vi "OSICS_FBL_Example.vi"() -> ()   [LabVIEW 2014, in "OSICS_LIB.lvlib"]
doc: "This example VI controls an OSICS Full Band Laser (FBL) remotely.\nAll commands and queries are sent to the OSICS SWT-APC, operating in \"Full-Band\" mode.\nThe OSICS mainframe can be connected via RS232 or GPIB."
uses:
  OSICS_LIB.lvlib
panel:
  out "Busy/Idle Status":bool
  in  "stop":bool
  in  "Laser State":bool
  in  "Power Unit":bool
  in  "WL/F unit":bool
  in  "VISA":refnum<visa-resource-name>="GPIB0::10::INSTR"
  in  "WL/Frequency Value":dbl format="%#_8g"
  in  "Power Value":dbl
  # "OSICS SWT-APC Full-Band Laser Example 1.1"
  # "l/¦"
  # "P"
  # "OSICS SWT-APC: Full-Band"
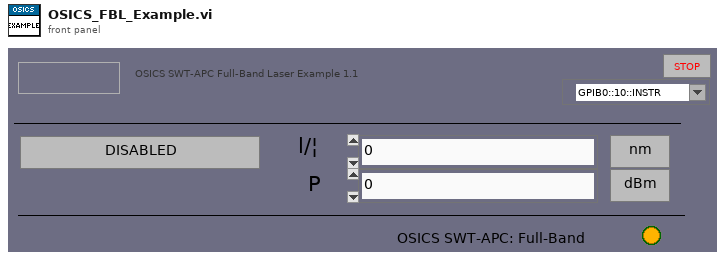
[diagram p1: front panel]
types:
  T1 = cluster{"Laser State":bool, "WL/F Value":dbl, "Power (dBm/mW)":dbl, "Power Limit":bool}
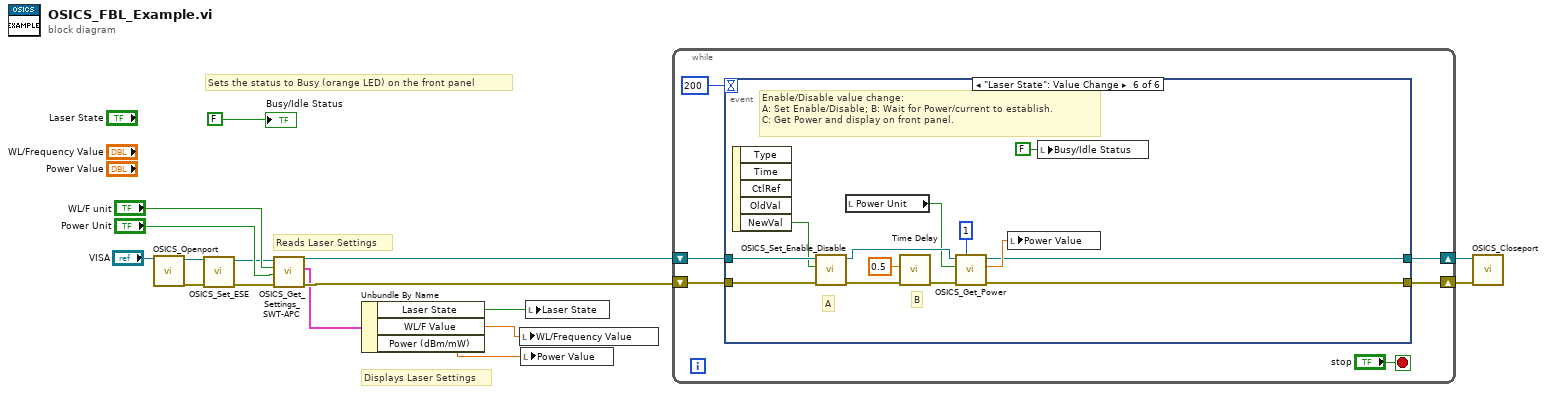
[diagram p0: block diagram]
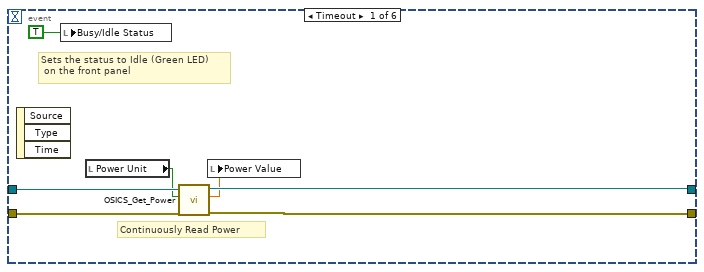
[diagram p2: hidden frame]
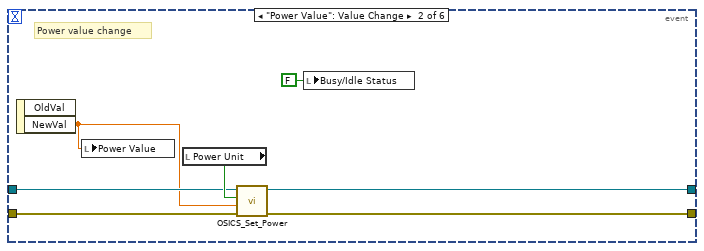
[diagram p3: hidden frame]
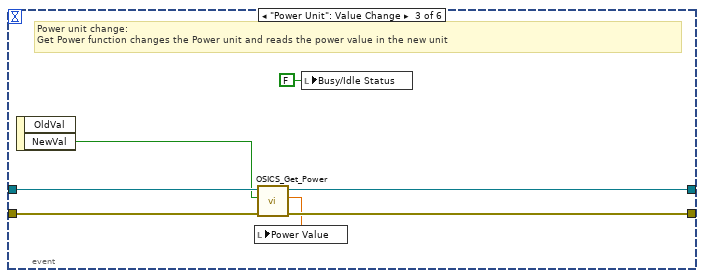
[diagram p4: hidden frame]
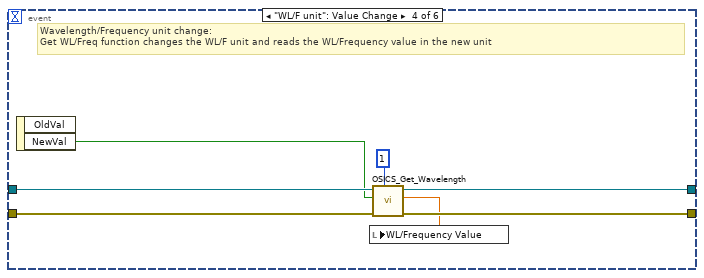
[diagram p5: hidden frame]
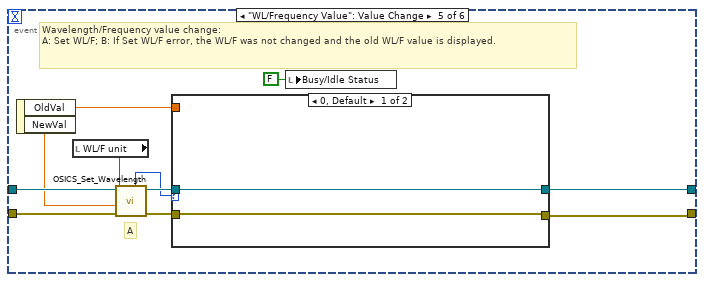
[diagram p6: hidden frame]
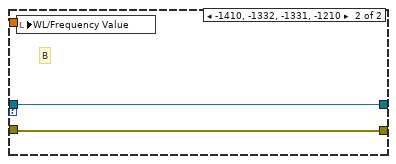
[diagram p7: hidden frame]
diagram:
  # "Sets the status to Busy (orange LED) on the front panel"
  # "Displays Laser Settings"
  # "Reads Laser Settings"
  n1 = call "OSICS_Openport.vi"("VISA IN"="VISA") -> ("error out"=w3:errorcluster, "VISA OUT"=w2:refnum<visa-resource-name>)  [unwired: 9 in]
  n2 = call "OSICS_Set_ESE.vi"("error in (no error)"=w3, "VISA resource name"=w2) -> ("error out"=w4:errorcluster, "VISA resource name out"=w1:refnum<visa-resource-name>)  [unwired: 8 in]
  n3 = call "OSICS_Get_Settings_SWT-APC.vi"("error in"=w4, "Power Unit(dBm/mW)"="Power Unit", "WL/F unit (nm/GHz)"="WL/F unit", "VISA IN"=w1) -> ("error out"=w10:errorcluster, "Laser Settings (Cluster)"=w6:T1, "VISA OUT"=w9:refnum<visa-resource-name>)  [unwired: 5 in]
  n4 = Unbundle By Name(w6) -> ("Laser State"=w11:bool, "WL/F Value"=w13:dbl, "Power (dBm/mW)"=w12:dbl)
  n5 = local write "WL/Frequency Value"(w13) -> ()
  n6 = local write "Power Value"(w12) -> ()
  n7 = local write "Laser State"(w11) -> ()
  n8 = while {
    shift-right: [w19] -> w16
    shift-left: w9 -> [w21]
    shift-right: [w18] -> w15
    shift-left: w10 -> [w20]
    stop <- "stop" stop-if-true
    n9 = event shown="[5] \"Laser State\": Value Change" {
      selector: _ -> [_ _ _ _ _ _]
      dyn-events: _ -> [_ _ _ _ _ _]
      timeout: 200 -> [_ _ _ _ _ _]
      tunnel: w21 -> [w29 w32 w43 w50 w61 w79]
      tunnel: w20 -> [w28 w33 w42 w48 w60 w78]
      tunnel: [w27 w36 w40 w46 w54 w68] -> w19
      tunnel: [w23 w34 w41 w47 w57 w70] -> w18
      event Timeout {
        # "Continuously Read Power"
        # "Sets the status to Idle (Green LED)\n on the front panel"
        n10 = event-data() -> ()  [unwired: 1 in, 3 out]
        n11 = local write "Busy/Idle Status"(TRUE ("Busy/Idle Status")) -> ()
        n12 = local read "Power Unit"() -> (w24:bool)
        n13 = call "OSICS_Get_Power.vi"("error in"=w28, "Power Unit(False: dBm)"=w24, "VISA IN"=w29) -> ("error out"=w23:errorcluster, "Power (dBm/mW)"=w25:dbl, "VISA OUT"=w27:refnum<visa-resource-name>)  [unwired: 4 in, 2 out]
        n14 = local write "Power Value"(w25) -> ()
      }
      event "Power Value": Value Change {
        # "Power value change"
        n15 = event-data() -> ("NewVal"=w30:dbl)  [unwired: 1 in, 1 out]
        n16 = local write "Power Value"(w30) -> ()
        n17 = local read "Power Unit"() -> (w35:bool)
        n18 = call "OSICS_Set_Power.vi"("error in"=w33, "P Value"=w30, "Power Unit(False:dBm)"=w35, "VISA IN"=w32) -> ("error out"=w34:errorcluster, "VISA OUT"=w36:refnum<visa-resource-name>)  [unwired: 5 in, 1 out]
        n19 = local write "Busy/Idle Status"(FALSE ("Busy/Idle Status")) -> ()
      }
      event "Power Unit": Value Change {
        # "Power unit change:\nGet Power function changes the Power unit and reads the power value in the new unit"
        n20 = event-data() -> ("NewVal"=w39:bool)  [unwired: 1 in, 1 out]
        n21 = call "OSICS_Get_Power.vi"("error in"=w42, "Power Unit(False: dBm)"=w39, "VISA IN"=w43) -> ("error out"=w41:errorcluster, "Power (dBm/mW)"=w38:dbl, "VISA OUT"=w40:refnum<visa-resource-name>)  [unwired: 4 in, 2 out]
        n22 = local write "Power Value"(w38) -> ()
        n23 = local write "Busy/Idle Status"(FALSE ("Busy/Idle Status")) -> ()
      }
      event "WL/F unit": Value Change {
        # "Wavelength/Frequency unit change:\nGet WL/Freq function changes the WL/F unit and reads the WL/Frequency value in the new unit"
        n24 = event-data() -> ("NewVal"=w49:bool)  [unwired: 1 in, 1 out]
        n25 = call "OSICS_Get_Wavelength.vi"("OSICS slot"=1, "error in"=w48, "WL/F unit (False:NM)"=w49, "VISA IN"=w50) -> ("error out"=w47:errorcluster, "WL/Frequency Value"=w45:dbl, "VISA OUT"=w46:refnum<visa-resource-name>)  [unwired: 4 in, 1 out]
        n26 = local write "WL/Frequency Value"(w45) -> ()
      }
      event "WL/Frequency Value": Value Change {
        # "A"
        # "Wavelength/Frequency value change:\nA: Set WL/F; B: If Set WL/F error, the WL/F was not changed and the old WL/F value is displayed."
        n27 = event-data() -> ("OldVal"=w58:dbl, "NewVal"=w59:dbl)  [unwired: 1 in]
        n28 = local read "WL/F unit"() -> (w53:bool)
        n29 = call "OSICS_Set_Wavelength.vi"("error in"=w60, "WL/Frequency Value"=w59, "WL/F unit (False:nm)"=w53, "VISA IN"=w61) -> ("error out"=w56:errorcluster, "VISA OUT"=w55:refnum<visa-resource-name>, "ERR"=w52:i32)  [unwired: 5 in]
        n30 = case shown="0, Default" w52 {
          tunnel: w58 -> [_ w66]
          tunnel: [w62 w65] -> w57
          tunnel: w56 -> [w62 w65]
          tunnel: w55 -> [w63 w64]
          tunnel: [w63 w64] -> w54
          frame 0, Default {
          }
          frame -1410, -1332, -1331, -1210 {
            # "B"
            n31 = local write "WL/Frequency Value"(w66) -> ()
          }
        }
        n32 = local write "Busy/Idle Status"(FALSE ("Busy/Idle Status")) -> ()
      }
      event "Laser State": Value Change {
        # "B"
        # "A"
        # "Enable/Disable value change:\nA: Set Enable/Disable; B: Wait for Power/current to establish.\nC: Get Power and display on front panel."
        n33 = event-data() -> ("NewVal"=w77:bool)  [unwired: 1 in, 4 out]
        n34 = call "OSICS_Set_Enable_Disable.vi"("error in"=w78, "Laser State (False:DISABLED)"=w77, "VISA IN"=w79) -> ("error out"=w76:errorcluster, "VISA OUT"=w73:refnum<visa-resource-name>)  [unwired: 6 in, 1 out]
        n35 = local read "Power Unit"() -> (w72:bool)
        n36 = call "Time Delay"("error in (no error)"=w76, "Delay Time (s)"=0.5) -> ("error out"=w75:errorcluster)  [unwired: 9 in]
        n37 = call "OSICS_Get_Power.vi"("OSICS slot"=1, "error in"=w75, "Power Unit(False: dBm)"=w72, "VISA IN"=w73) -> ("error out"=w70:errorcluster, "Power (dBm/mW)"=w71:dbl, "VISA OUT"=w68:refnum<visa-resource-name>)  [unwired: 3 in, 2 out]
        n38 = local write "Power Value"(w71) -> ()
        n39 = local write "Busy/Idle Status"(FALSE ("Busy/Idle Status")) -> ()
      }
    }
  }
  n40 = call "OSICS_Closeport.vi"("error in"=w15, "VISA IN"=w16) -> ()  [unwired: 9 in, 1 out]
  "Busy/Idle Status" <- FALSE ("Busy/Idle Status")
